vi "act-0020-3-en.vi"() -> ()   [LabVIEW 2010]
uses:
  support/lv_07.lvlib
panel:
  in  "Pu":dbl
  out "Qe":dbl
  in  "Qa":dbl
  out "Cc init":dbl
  out "Ccpc nv":dbl
  in  "Cc":dbl
  in  "T":dbl
  in  "Ccpc":dbl
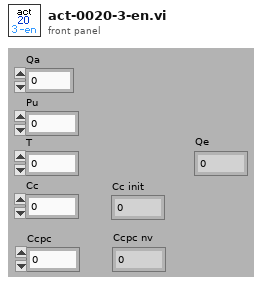
[diagram p1: front panel]
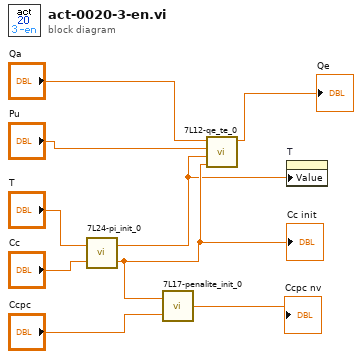
[diagram p0: block diagram]
diagram:
  n1 = call "7L24-pi_init_0.vi"("Cc"="Cc", "T"="T") -> ("Cc init"=w3:dbl, "T init"=w1:dbl)
  "Cc init" <- w3
  n2 = call "7L17-penalite_init_0.vi"("Ccpc"="Ccpc", "Cc"=w3) -> ("Ccpc init"=→"Ccpc nv":dbl)
  n3 = call "7L12-qe_te_0.vi"("Cc"=w3, "T"=w1, "Pu"="Pu", "Qa"="Qa") -> ("Qe"=→"Qe":dbl)  [unwired: 5 in, 2 out]
  n4 = property on="T" class="NumDig (strict)"("Value"=w1) -> ()  [unwired: 2 in, 2 out]
